vi "CreateBanksNode.vi"(7 "DOM Document":refnum<k20>, 8 "Error In":errorcluster, 11 "Banks":T1[](array[typedef])) -> (0 "Error Out":errorcluster, 3 "Banks Node":refnum<k20>)   [LabVIEW 2012]
uses:
  BankConfiguration.ctl
  libs/LV-Utilities/LV-Utilities.lvlib
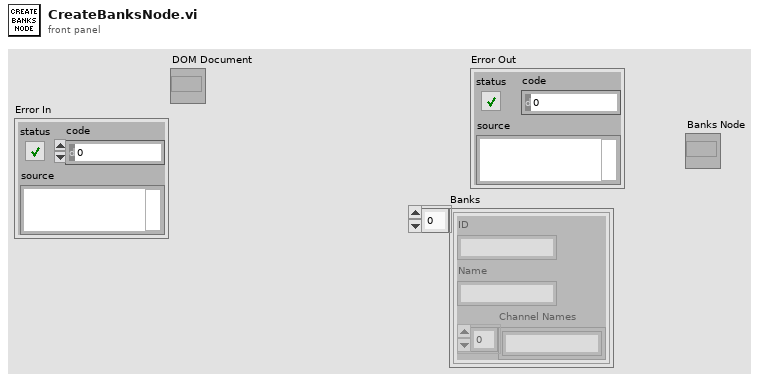
[diagram p1: front panel]
types:
  T1 = typedef "BankConfiguration.ctl" = cluster{"ID":string, "Name":string, "Channel Names":string[]}
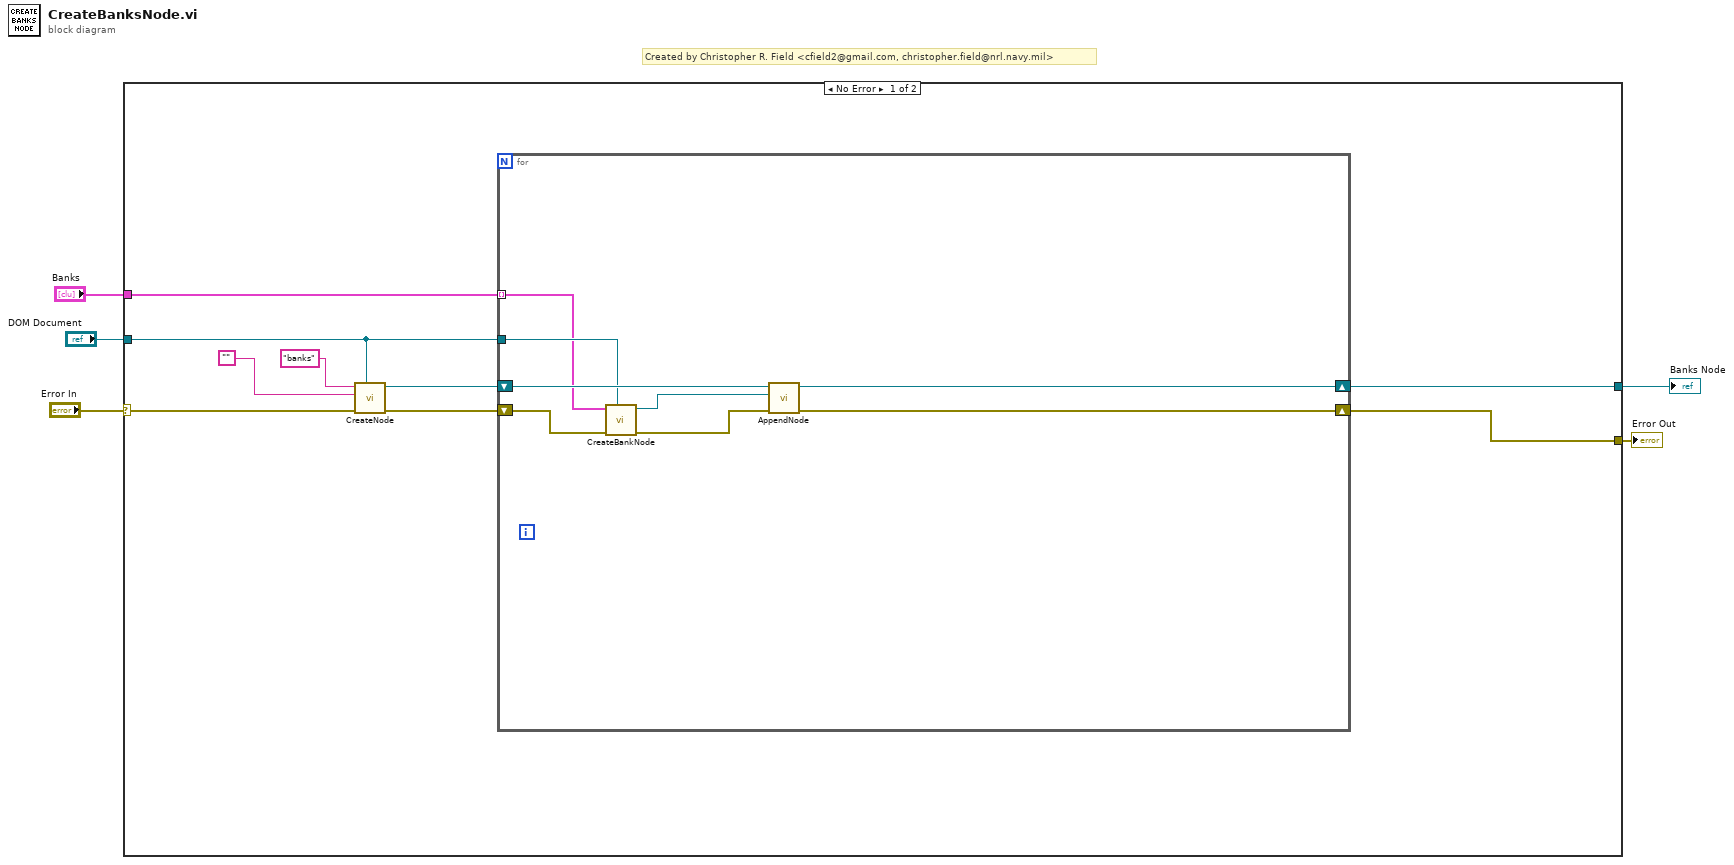
[diagram p0: block diagram]
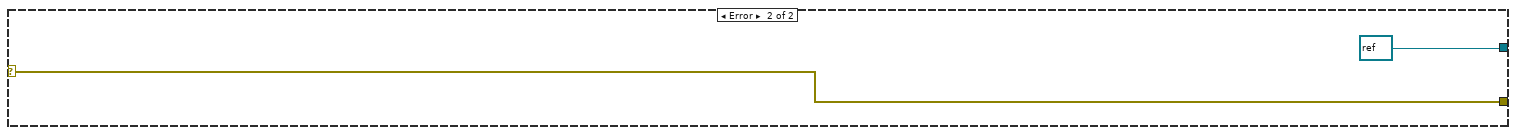
[diagram p2: hidden frame]
diagram:
  # "Created by Christopher R. Field <cfield2@gmail.com, christopher.field@nrl.navy.mil>"
  n1 = case shown="No Error" "Error In" {
    selector: "Error In" -> [w14 w24]
    tunnel: "DOM Document" -> [w9 _]
    tunnel: [w8 refnum<k20> refnum ("Channel Node 2")] -> w2
    tunnel: [w7 w24] -> w3
    tunnel: "Banks" -> [w6 _]
    frame No Error {
      n2 = call "CreateNode.vi"("DOM Document"=w9, "Error In"=w14, "Text"="", "Tag Name"="banks") -> ("Error out"=w13:errorcluster, "Node"=w10:refnum<k20>)  [unwired: 6 in]
      n3 = for {
        tunnel: w6 -> [w18] mode=indexing
        shift-right: [w20] -> w7
        shift-left: w13 -> [w17]
        shift-right: [w21] -> w8
        shift-left: w10 -> [w22]
        tunnel: w9 -> [w19]
        n4 = call "CreateBankNode.vi"("DOM Document"=w19, "Error In"=w17, "Bank Configuration"=w18) -> ("Error Out"=w16:errorcluster, "Bank Channel Node"=w15:refnum<k20>)  [unwired: 7 in]
        n5 = call "AppendNode.vi"("Error In"=w16, "Child Node"=w15, "Parent Node In"=w22) -> ("Error Out"=w20:errorcluster, "Parent Node Out"=w21:refnum<k20>)  [unwired: 7 in]
      }
    }
    frame Error {
    }
  }
  "Error Out" <- w3
  "Banks Node" <- w2
